vi "Set Needle Valve.vi"(8 "error in (no error)":errorcluster, 10 "Needle Valve (%)":dbl min=0.0 max=100.0, 11 "Instrument.1820 in":refnum<class "Instrument.Oxford1820.lvclass">) -> (0 "error out":errorcluster, 2 "Response":string, 3 "Instrument.1820 in":refnum<class "Instrument.Oxford1820.lvclass">)   [LabVIEW 2019, in "Instrument.Oxford1820.lvclass"]
uses:
  Instrument.Oxford1820.lvclass
  Typedefs/Instrument.Oxford1820.protectedCommands-enum.ctl
  31e74666-4a62-4e3e-81a3-d19e0cd87890.vi/20e622f4-2d6d-4c52-af8b-83e24b17d302.vi
  31e74666-4a62-4e3e-81a3-d19e0cd87890.vi/cf2cdd97-1106-4a1c-ad30-e60bf5142a67.vi
  <vilib>/Utility/Data Type/Get Type Information.vi
  <vilib>/JDP Science/JSONtext/JSON text to Variant.vi
  <vilib>/JDP Science/JSONtext/LVClass Serializer/JSONtext LVClass Serializer.lvclass
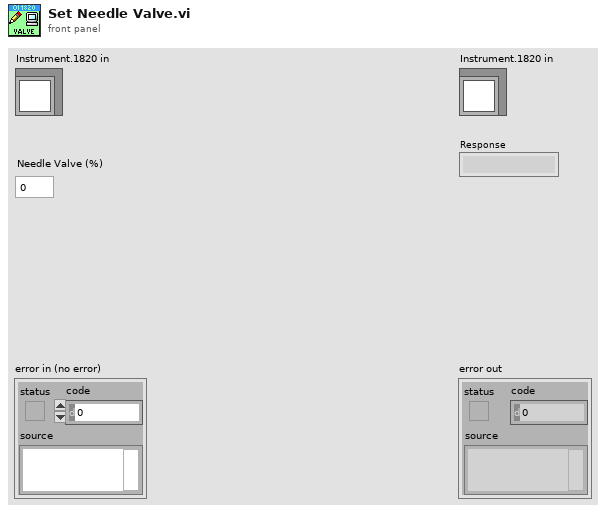
[diagram p1: front panel]
types:
  T1 = typedef "Instrument.Oxford1820.lvclass/Instrument.Oxford1820.protectedCommands-enum.ctl" = enum16{"Hold", "RampToSet", "RampToZero", "Clamp", "setTarget", "setSwitchHeat", "setLambda", "setFillMode", "setNeedleValve", "getStatus", "getTarget", "getSwitchHeat", "getPSUField", "setSequenceStatus"}
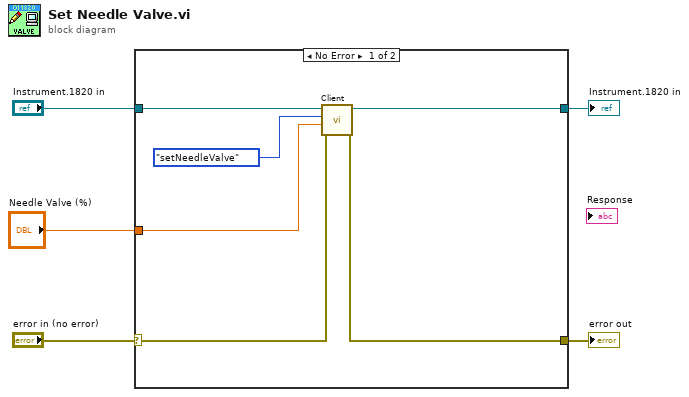
[diagram p0: block diagram]
diagram:
  n1 = case shown="No Error" "error in (no error)" {
    selector: "error in (no error)" -> [w11 w13]
    tunnel: [w6 w13] -> w4
    tunnel: [w7 w12] -> w2
    tunnel: "Instrument.1820 in" -> [w8 w12]
    tunnel: "Needle Valve (%)" -> [w10 _]
    frame No Error {
      n2 = call-dynamic "Client.vi"("error in (no error)"=w11, "Data in"=w10, "Command in"=Instrument.Oxford1820.protectedCommands-enum."setNeedleValve" ("Commands"), "Instrument in"=w8) -> ("error out"=w6:errorcluster, "Instrument out"=w7:refnum<class "Instrument.Oxford1820.lvclass">)  [unwired: 4 in, 2 out]
    }
    frame Error {
    }
  }
  "error out" <- w4
  "Instrument.1820 in" <- w2
